vi "Array SV Count.vi"(8 "Error In":errorcluster, 10 "Initial number":i32, 11 "Type array":string[](array[string])) -> (0 "Error Out":errorcluster, 2 "Number of scalar SV":i32)   [LabVIEW 2014]
doc: "This VI counts the number of scalar shared variables."
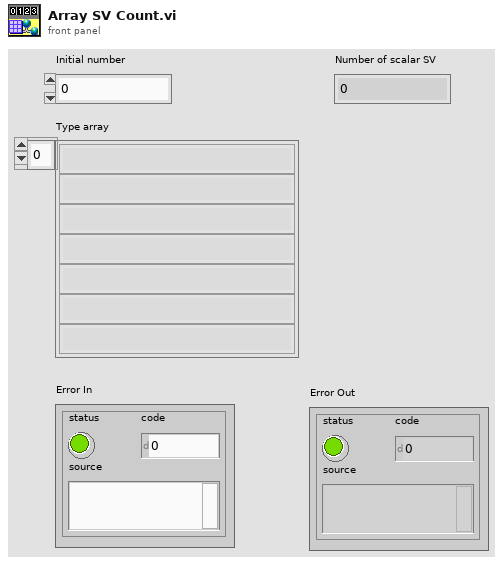
[diagram p1: front panel]
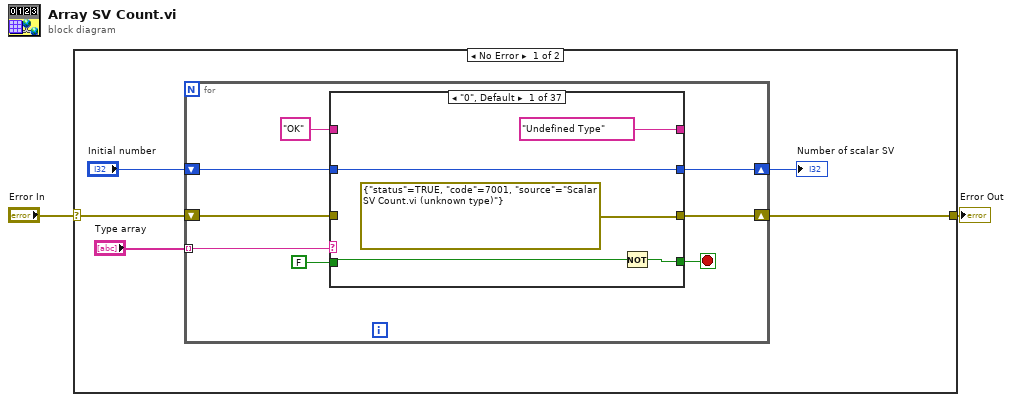
[diagram p0: block diagram]
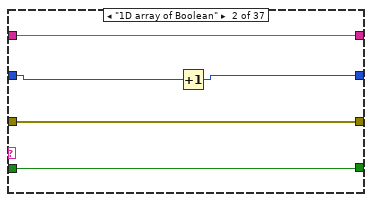
[diagram p2: hidden frame]
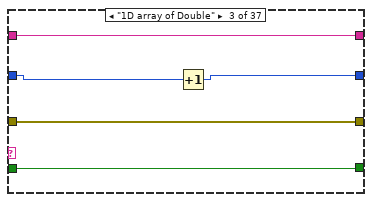
[diagram p3: hidden frame]
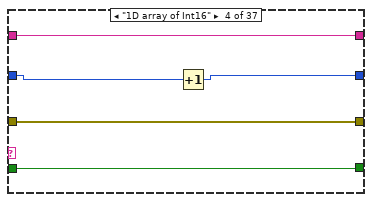
[diagram p4: hidden frame]
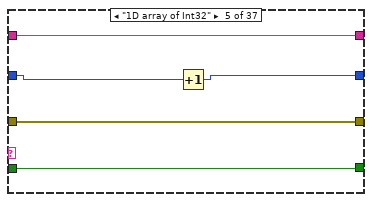
[diagram p5: hidden frame]
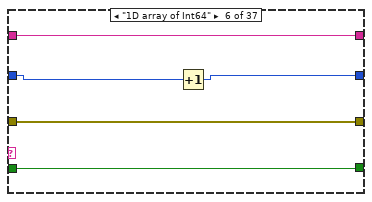
[diagram p6: hidden frame]
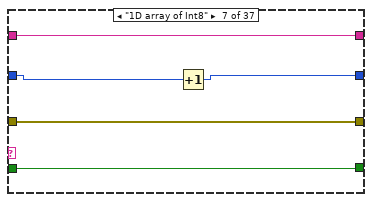
[diagram p7: hidden frame]
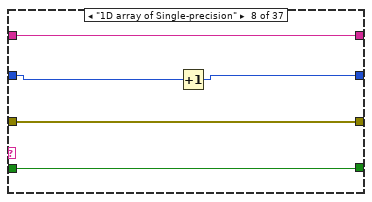
[diagram p8: hidden frame]
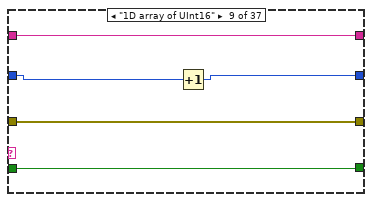
[diagram p9: hidden frame]
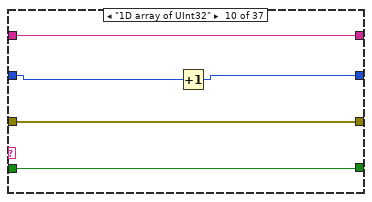
[diagram p10: hidden frame]
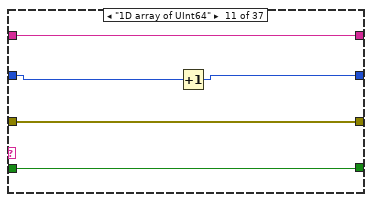
[diagram p11: hidden frame]
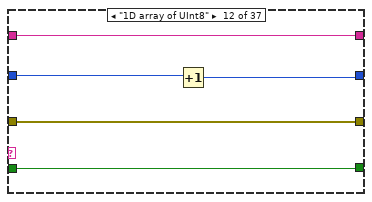
[diagram p12: hidden frame]
diagram:
  n1 = case shown="No Error" "Error In" {
    selector: "Error In" -> [w7 w176]
    tunnel: [w6 w176] -> w1
    frame No Error {
      n2 = for {
        shift-right: [w14] -> w6
        shift-left: w7 -> [w15]
        tunnel: "Type array" -> [w10] mode=indexing
        shift-right: [w8] -> w3
        shift-left: "Initial number" -> [w9]
        stop <- w11 stop-if-true
        n3 = case shown="\"0\", Default" w10 {
          tunnel: w15 -> [_ w23 w28 w33 w38 w43 w48 w53 w58 w63 w68 w73 w76 w80 w84 w88 w92 w96 w100 w104 w108 w112 w116 w121 w125 w129 w133 w137 w141 w145 w149 w154 w157 w161 w165 w169 w173]
          tunnel: [errorcluster {"status"=TRUE, "code"=7001, "source"="Scalar SV Count.vi (unknown type)"} ("error constant") w23 w28 w33 w38 w43 w48 w53 w58 w63 w68 w73 w76 w80 w84 w88 w92 w96 w100 w104 w108 w112 w116 w121 w125 w129 w133 w137 w141 w145 w149 w154 w157 w161 w165 w169 w173] -> w14
          tunnel: ["Undefined Type" w25 w30 w35 w40 w45 w50 w55 w60 w65 w70 w75 w79 w83 w87 w91 w95 w99 w103 w107 w111 w115 w119 w123 w127 w131 w135 w139 w143 w147 w151 w155 w159 w163 w167 w171 w175] -> _
          tunnel: "OK" -> [_ w25 w30 w35 w40 w45 w50 w55 w60 w65 w70 w75 w79 w83 w87 w91 w95 w99 w103 w107 w111 w115 w119 w123 w127 w131 w135 w139 w143 w147 w151 w155 w159 w163 w167 w171 w175]
          tunnel: FALSE -> [w19 w24 w29 w34 w39 w44 w49 w54 w59 w64 w69 w74 w78 w82 w86 w90 w94 w98 w102 w106 w110 w114 w118 w122 w126 w130 w134 w138 w142 w146 w150 w153 w158 w162 w166 w170 w174]
          tunnel: [w18 w24 w29 w34 w39 w44 w49 w54 w59 w64 w69 w74 w78 w82 w86 w90 w94 w98 w102 w106 w110 w114 w118 w122 w126 w130 w134 w138 w142 w146 w150 w153 w158 w162 w166 w170 w174] -> w11
          tunnel: w9 -> [w16 w22 w27 w32 w37 w42 w47 w52 w57 w62 w67 w72 w77 w81 w85 w89 w93 w97 w101 w105 w109 w113 w117 w120 w124 w128 w132 w136 w140 w144 w148 w152 w156 w160 w164 w168 w172]
          tunnel: [w16 w21 w26 w31 w36 w41 w46 w51 w56 w61 w66 w71 w77 w81 w85 w89 w93 w97 w101 w105 w109 w113 w117 w120 w124 w128 w132 w136 w140 w144 w148 w152 w156 w160 w164 w168 w172] -> w8
          frame "0", Default {
            n4 = Not(x=w19) -> (.not. x?=w18:bool)
          }
          frame "1D array of Boolean" {
            n5 = Increment(x=w22) -> (x+1=w21:i32)
          }
          frame "1D array of Double" {
            n6 = Increment(x=w27) -> (x+1=w26:i32)
          }
          frame "1D array of Int16" {
            n7 = Increment(x=w32) -> (x+1=w31:i32)
          }
          frame "1D array of Int32" {
            n8 = Increment(x=w37) -> (x+1=w36:i32)
          }
          frame "1D array of Int64" {
            n9 = Increment(x=w42) -> (x+1=w41:i32)
          }
          frame "1D array of Int8" {
            n10 = Increment(x=w47) -> (x+1=w46:i32)
          }
          frame "1D array of Single-precision" {
            n11 = Increment(x=w52) -> (x+1=w51:i32)
          }
          frame "1D array of UInt16" {
            n12 = Increment(x=w57) -> (x+1=w56:i32)
          }
          frame "1D array of UInt32" {
            n13 = Increment(x=w62) -> (x+1=w61:i32)
          }
          frame "1D array of UInt64" {
            n14 = Increment(x=w67) -> (x+1=w66:i32)
          }
          frame "1D array of UInt8" {
            n15 = Increment(x=w72) -> (x+1=w71:i32)
          }
          frame "2D array of Boolean" {
          }
          frame "2D array of Double" {
          }
          frame "2D array of Int16" {
          }
          frame "2D array of Int32" {
          }
          frame "2D array of Int64" {
          }
          frame "2D array of Int8" {
          }
          frame "2D array of Single-precision" {
          }
          frame "2D array of UInt16" {
          }
          frame "2D array of UInt32" {
          }
          frame "2D array of UInt64" {
          }
          frame "2D array of UInt8" {
          }
          frame "Boolean" {
          }
          frame "String" {
          }
          frame "Double" {
          }
          frame "Fixed Point - signed" {
          }
          frame "Fixed Point - unsigned" {
          }
          frame "Int16" {
          }
          frame "Int32" {
          }
          frame "Int64" {
          }
          frame "Int8" {
          }
          frame "Single-precision" {
          }
          frame "UInt16" {
          }
          frame "UInt32" {
          }
          frame "UInt64" {
          }
          frame "UInt8" {
          }
        }
      }
      "Number of scalar SV" <- w3
    }
    frame Error {
    }
  }
  "Error Out" <- w1
